vi "LibXML_ReplaceAttributeValue.vi"(6 "New Value":string, 8 "error in":errorcluster, 9 "attr. name":string="/ScanMaster/Devices/Device/description", 10 "xpathexpr (root)":string="/ScanMaster/Devices/Device/description", 11 "doc":u32) -> (0 "error out":errorcluster, 3 "doc copy out":u32)   [LabVIEW 2019, in "Tools.lvlib" / "LibXML.lvlib"]
doc: "Replaces the value of an attribute at the xpathexpr with the attribute name and new value specified"
uses:
  LibXML.lvlib
  Error Cluster From Error Code_subroutine.vi
  <vilib>/Utility/error.llb/Trim Whitespace.vi
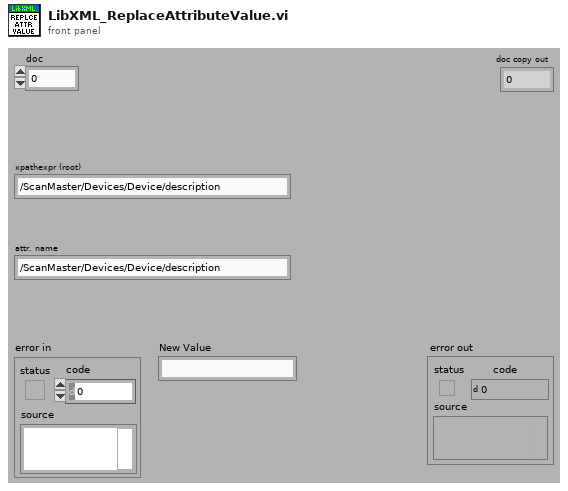
[diagram p1: front panel]
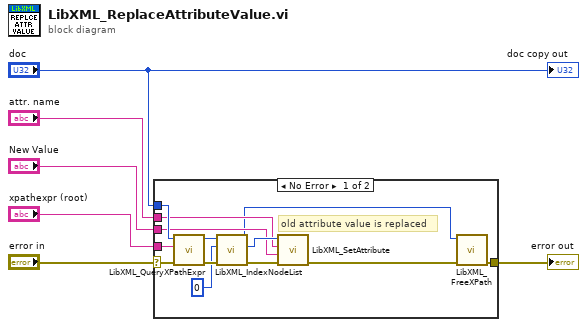
[diagram p0: block diagram]
diagram:
  n1 = case shown="No Error" "error in" {
    selector: "error in" -> [w7 w20]
    tunnel: "xpathexpr (root)" -> [w19 _]
    tunnel: "doc" -> [w18 _]
    tunnel: [w17 w20] -> w4
    tunnel: "attr. name" -> [w12 _]
    tunnel: "New Value" -> [w11 _]
    frame No Error {
      # "old attribute value is replaced"
      n2 = call "LibXML_QueryXPathExpr.vi"("error in"=w7, "XPathExpr"=w19, "doc"=w18) -> ("error out"=w16:errorcluster, "xmlXPathObj"=w8:u32)  [unwired: 7 in]
      n3 = call "LibXML_IndexNodeList.vi"("error in"=w16, "index"=0, "XPathObj"=w8) -> ("error out"=w14:errorcluster, "NodePtr"=w13:u32, "XPathObj out"=w9:u32)  [unwired: 6 in]
      n4 = call "LibXML_SetAttribute.vi"("error in"=w14, "value"=w11, "name"=w12, "node"=w13) -> ("error out"=w10:errorcluster)  [unwired: 6 in, 1 out]
      n5 = call "LibXML_FreeXPath.vi"("error in"=w10, "XPathObj"=w9) -> ("error out"=w17:errorcluster)  [unwired: 9 in]
    }
    frame Error {
    }
  }
  "error out" <- w4
  "doc copy out" <- "doc"
